vi "Compile FIU.vi"(8 "error in (no error)":errorcluster, 11 "Device Item Ref in":T5 format="%.0x") -> (0 "error out":errorcluster, 1 "FIU Engine Data":T1 {"Ordered Channels" format="%.0x"; "RT IDs"."Slot #" max=15; "RT IDs"."Chip Address (A2 A1 A0)" max=7}, 2 "Initial FIU SPI CMDs":u64[](array[numeric]), 3 "Device Item Ref out":T5 format="%.0x")   [LabVIEW 2014, in "SLSC configuration System Explorer.lvlib"]
uses:
  SLSC configuration System Explorer.lvlib
  <vilib>/NI Veristand/Custom Device API/Custom Device Item Ref.ctl
  Shared/Type Defs/RT Engine Data.ctl
  Shared/Type Defs/RT IDs.ctl
  Shared/SPI Utility/Slot #.ctl
  Shared/MCP23S17/Chip Address.ctl
  Shared/Constants.vi
  <vilib>/NI Veristand/Custom Device API/Get Item Property (U16).vi
  <vilib>/NI Veristand/Custom Device Tools/Custom Device Utility Library/Custom Device Utility Library.lvlib
  Shared/SLSC configuration Shared.lvlib
  <vilib>/NI Veristand/Custom Device API/Custom Device API.lvlib
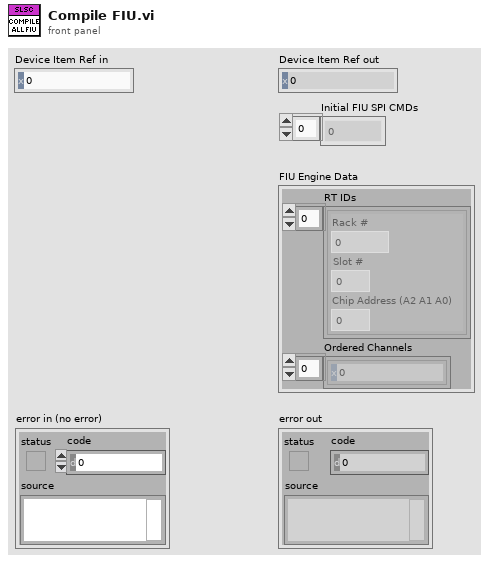
[diagram p1: front panel]
types:
  T1 = typedef "SLSC configuration Shared.lvlib/RT Engine Data.ctl" = cluster{"RT IDs":T2[], "Ordered Channels":T5[]}
  T2 = typedef "SLSC configuration Shared.lvlib/RT IDs.ctl" = cluster{"Rack #":u8, "Slot #":T3, "Chip Address (A2 A1 A0)":T4}
  T3 = typedef "SLSC configuration Shared.lvlib/Slot #.ctl" = u8
  T4 = typedef "SLSC configuration Shared.lvlib/Chip Address.ctl" = u8
  T5 = typedef "Custom Device API.lvlib/Custom Device Item Ref.ctl" = u64
  T6 = typedef "SLSC configuration Shared.lvlib/Fault State.ctl" = enum8{"No Fault Output 1", "Open Circuit 100 Hz", "Ground 100 Hz", "Open Circuit", "Ground", "Fail Rail 1", "Fail Rail 2", "No Fault Output 2"}
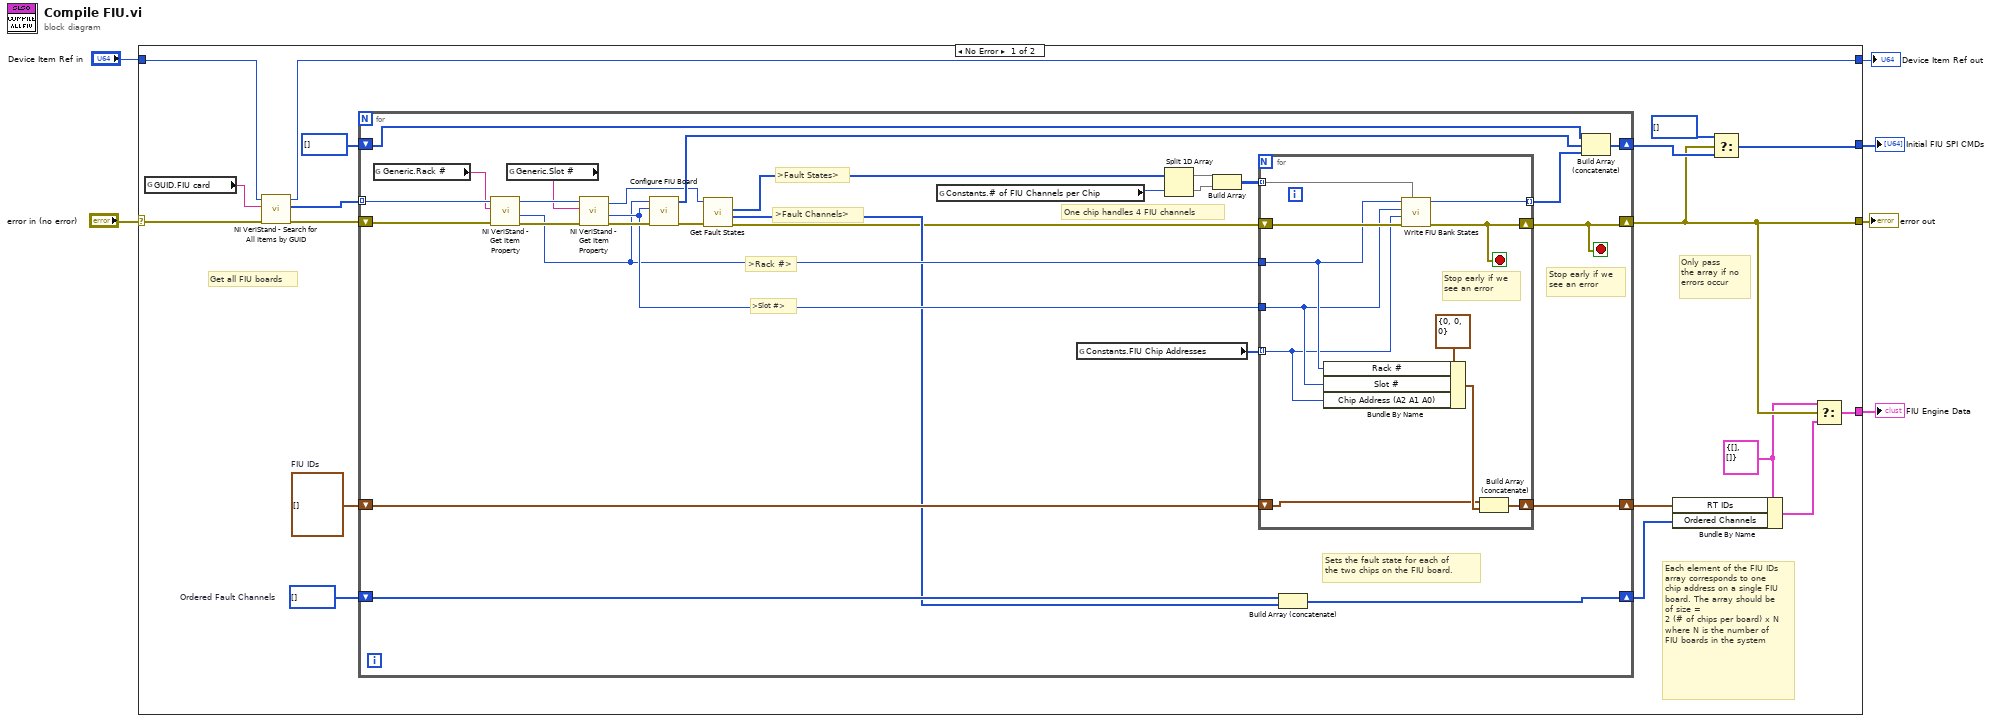
[diagram p0: block diagram]
diagram:
  n1 = case shown="No Error" "error in (no error)" {
    selector: "error in (no error)" -> [w21 w65]
    tunnel: [w10 w65] -> w6
    tunnel: "Device Item Ref in" -> [w15 w64]
    tunnel: [w7 _] -> w3
    tunnel: [w11 _] -> w2
    tunnel: [w14 w64] -> w1
    frame No Error {
      w9 = T1 {"RT IDs"=[], "Ordered Channels"=[]} ("FIU Engine Data")
      w18 = T5[] []  # Ordered Fault Channels
      w19 = T2[] []  # FIU IDs
      # "Only pass\nthe array if no\nerrors occur"
      # "Get all FIU boards"
      # "Each element of the FIU IDs array corresponds to one chip address on a single FIU board. The array should be of size =\n2 (# of chips per board) x N where N is the number of FIU boards in the system"
      n2 = global read "Constants.vi" "GUID.FIU card"() -> (w24:string)
      n3 = call <vilib>:"NI VeriStand - Search for All Items by GUID.vi"("error in"=w21, "Item GUID"=w24, "Section Ref in"=w15) -> ("error out"=w23:errorcluster, "Item Refs"=w22:T5[], "Section Ref out"=w14:T5)  [unwired: 5 in, 1 out]
      n4 = for {
        tunnel: w22 -> [w51] mode=indexing
        shift-right: [w30] -> w10
        shift-left: w23 -> [w52]
        shift-right: [w39] -> w13
        shift-left: u64[] [] ("SPI FIFO Messages") -> [w45]
        shift-right: [w36] -> w17
        shift-left: w19 -> [w37]
        shift-right: [w34] -> w16
        shift-left: w18 -> [w35]
        stop <- w30 stop-if-true
        # "Stop early if we\nsee an error"
        # "One chip handles 4 FIU channels"
        # ">Fault States>"
        # ">Fault Channels>"
        # "Sets the fault state for each of\nthe two chips on the FIU board."
        # ">Slot #>"
        # ">Rack #>"
        n5 = global read "Constants.vi" "Generic.Rack #"() -> (w50:string)
        n6 = call-poly <vilib>:"NI VeriStand - Get Item Property.vi"("error in (no error)"=w52, "Property Name"=w50, "Item Ref in"=w51) -> ("error out"=w49:errorcluster, "Value"=w38:u16, "Item Ref out"=w48:T5)  [unwired: 5 in, 1 out]
        n7 = global read "Constants.vi" "Generic.Slot #"() -> (w47:string)
        n8 = call-poly <vilib>:"NI VeriStand - Get Item Property.vi"("error in (no error)"=w49, "Property Name"=w47, "Item Ref in"=w48) -> ("error out"=w46:errorcluster, "Value"=w41:u16, "Item Ref out"=w42:T5)  [unwired: 5 in, 1 out]
        n9 = call "Configure FIU Board.vi"("error in (no error)"=w46, "Slot #"=w41, "Rack #"=w38) -> ("error out"=w43:errorcluster, "SPI FIFO Messages"=w44:u64[])  [unwired: 7 in]
        n10 = call "Get Fault States.vi"("error in (no error)"=w43, "FIU Board Ref in"=w42) -> ("error out"=w31:errorcluster, "Ordered Fault Channels"=w32:T5[], "Fault States"=w33:T6[])  [unwired: 6 in, 1 out]
        n11 = global read "Constants.vi" "Constants.# of FIU Channels per Chip"() -> (w25:u8)
        n12 = global read "Constants.vi" "Constants.FIU Chip Addresses"() -> (w26:u8[])
        n13 = Split 1D Array(array=w33, index=w25) -> (first subarray=w29:T6[], second subarray=w28:T6[])
        n14 = Build Array(w29, w28) -> (w27:T6[][])
        n15 = for {
          tunnel: w26 -> [w58] mode=indexing
          shift-right: [w53] -> w30
          shift-left: w31 -> [w63]
          tunnel: w41 -> [w59]
          tunnel: w38 -> [w60]
          tunnel: [w62] -> w40 mode=indexing
          shift-right: [w55] -> w36
          shift-left: w37 -> [w56]
          tunnel: w27 -> [w54] mode=indexing
          stop <- w53 stop-if-true
          # "Stop early if we\nsee an error"
          n16 = Bundle By Name(cluster=T2 {"Rack #"=0, "Slot #"=0, "Chip Address (A2 A1 A0)"=0}, "Rack #"=w60, "Slot #"=w59, "Chip Address (A2 A1 A0)"=w58) -> (w57:T2)
          n17 = call "Write FIU Bank States.vi"("Fault States"=w54, "error in (no error)"=w63, "Chip Address (A2 A1 A0)"=w58, "Slot #"=w59, "Rack #"=w60) -> ("error out"=w53:errorcluster, "FIFO SPI Message"=w62:u64)  [unwired: 4 in, 1 out]
          n18 = Build Array (concatenate)(w56, w57) -> (w55:T2[])
        }
        n19 = Build Array (concatenate)(w35, w32) -> (w34:T5[])
        n20 = Build Array (concatenate)(w45, w44, w40) -> (w39:u64[])
      }
      n21 = Bundle By Name(cluster=w9, "RT IDs"=w17, "Ordered Channels"=w16) -> (w8:T1)
      n22 = Select(t=u64[] [], s=w10, f=w13) -> (s? t:f=w11:u64[])
      n23 = Select(t=w9, s=w10, f=w8) -> (s? t:f=w7:T1)
    }
    frame Error {
    }
  }
  "error out" <- w6
  "Device Item Ref out" <- w1
  "FIU Engine Data" <- w3
  "Initial FIU SPI CMDs" <- w2
